vi "Workspace.Initialize.vi"(11 "State":T1) -> (0 "error out":errorcluster, 3 "State":T1)   [LabVIEW 2023, in "J1939 Workspace Shared.lvlib"]
uses:
  J1939 Workspace Shared.lvlib
  Types/UI.StateVariables.ctl
  <vilib>/NI VeriStand/Display Template Support/DisplayTemplateSupport.llb/enum_Display Template Handler Minimal To Widget Msg.ctl
  <vilib>/NI VeriStand/Execution/Workspace/SystemStateRegEventRef.ctl
  <vilib>/NI VeriStand/Execution/Workspace/Target State Info.ctl
  <vilib>/NI VeriStand/Execution/Workspace/Target State.ctl
  Types/Private Data.ctl
  <vilib>/NI/STM/TCP/TCP Connection Info.ctl
  <vilib>/NI/STM/SubVIs/MetaDataElement.ctl
  Addon/Addon Shared/Types/Error Cluster.ctl
  Addon/Addon Shared/Types/Error Types.ctl
  NationalInstruments.VeriStand.SystemStorage
  <vilib>/NI VeriStand/Display Template Support/DisplayTemplateSupport.llb/enum_Display Template Handler Minimal To Workspace.ctl
  <vilib>/NI VeriStand/Execution/Workspace/WorkspaceAPI.ctl
  NationalInstruments.VeriStand.ClientAPI
  <vilib>/NI VeriStand/Execution/Workspace/SystemStateEventRef.ctl
  Types/UI.Refs.ctl
  SubModules/CAN-Streaming-Support/Source/Addon/Addon Shared/Types/Type Filter.ctl
  SubModules/CAN-Streaming-Support/Source/Addon/Addon Shared/Types/Direction Filter.ctl
  SubModules/CAN-Streaming-Support/Source/UIs/Workspace Shared/Types/Host Stream Queue Refs.ctl
  SubModules/CAN-Streaming-Support/Source/UIs/Workspace Shared/Types/Host Stream Queue Type.ctl
  SubModules/CAN-Streaming-Support/Source/UIs/Workspace Shared/Types/Host Stream Queue Command.ctl
  <vilib>/xnet/xnet.llb/XNET Frame CAN.ctl
  <vilib>/xnet/xnet.llb/XNET Frame Type CAN.ctl
  <vilib>/NI VeriStand/Execution/Workspace/NI_VS Workspace ExecutionAPI.lvlib
  Addon/Addon Shared/J1939 Addon Shared.lvlib
  SubModules/CAN-Streaming-Support/Source/UIs/Workspace Shared/CAN Stream Support Workspace Shared.lvlib
  <vilib>/NI/STM/NI STM.lvlib
  SubModules/CAN-Streaming-Support/Source/Addon/Addon Shared/CAN Stream Support Shared.lvlib
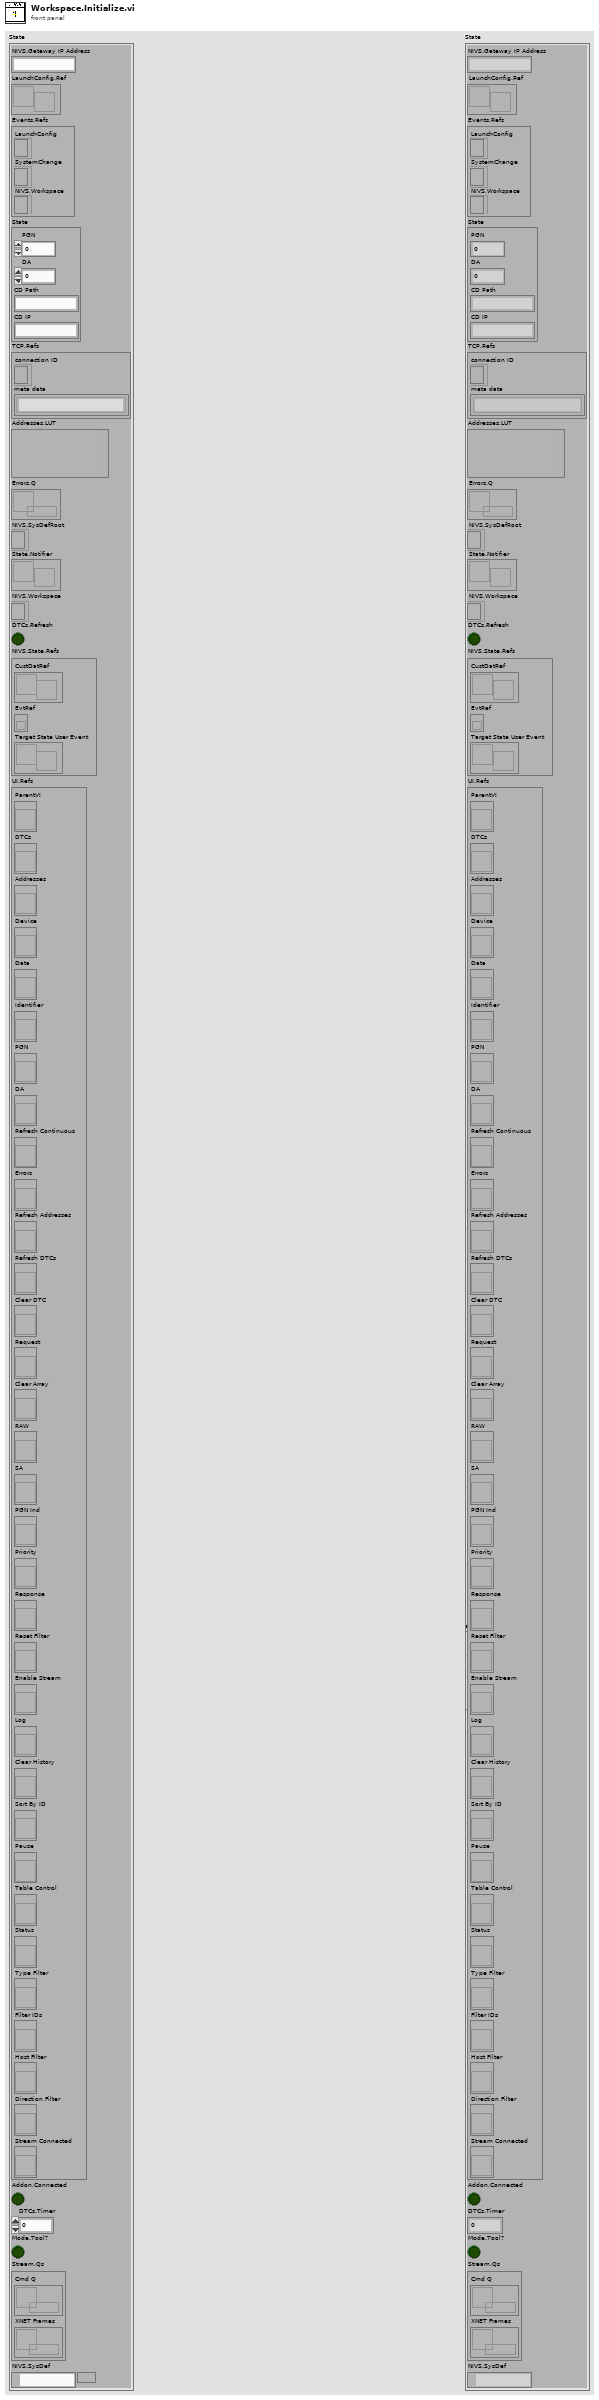
[diagram p1: front panel]
types:
  T1 = typedef "J1939 Workspace Shared.lvlib/UI.StateVariables.ctl" = cluster{"NIVS.Gateway IP Address":string, "LaunchConfig.Ref":refnum<user-event>, "Events.Refs":cluster{"LaunchConfig":refnum<event-registration>, "SystemChange":T2, "NIVS.Workspace":refnum<event-registration>}, "State":T3, "TCP.Refs":T4, "Addresses.LUT":variant, "Errors.Q":refnum<queue>, "NIVS.SysDefRoot":refnum<k24>, "State.Notifier":refnum<user-event>, "NIVS.Workspace":T6, "DTCs.Refresh":bool, "NIVS.State.Refs":T7, "UI.Refs":T8, "Addon.Connected":bool, "DTCs.Timer":u32, "Mode.Tool?":bool, "Stream.Qs":T9, "NIVS.SysDef":path}
  T2 = typedef "NI_VS Workspace ExecutionAPI.lvlib/SystemStateRegEventRef.ctl" = refnum<event-registration>
  T3 = typedef "J1939 Workspace Shared.lvlib/Private Data.ctl" = cluster{"PGN":u32, "DA":u8, "CD Path":string, "CD IP":string}
  T4 = typedef "NI STM.lvlib/TCP Connection Info.ctl" = cluster{"connection ID":refnum<k5>, "meta data":T5[]}
  T5 = typedef "NI STM.lvlib/MetaDataElement.ctl" = string
  T6 = typedef "NI_VS Workspace ExecutionAPI.lvlib/WorkspaceAPI.ctl" = refnum<k24>
  T7 = typedef "NI_VS Workspace ExecutionAPI.lvlib/SystemStateEventRef.ctl" = cluster{"CustDatRef":refnum<user-event>, "EvtRef":refnum<k27>, "Target State User Event":refnum<user-event>}
  T8 = typedef "J1939 Workspace Shared.lvlib/UI.Refs.ctl" = cluster{"ParentVI":refnum<vi>, "DTCs":refnum<vi>, "Addresses":refnum<vi>, "Device":refnum<vi>, "Data":refnum<vi>, "Identifier":refnum<vi>, "PGN":refnum<vi>, "DA":refnum<vi>, "Refresh Continuous":refnum<vi>, "Errors":refnum<vi>, "Refresh Addresses":refnum<vi>, "Refresh DTCs":refnum<vi>, "Clear DTC":refnum<vi>, "Request":refnum<vi>, "Clear Array":refnum<vi>, "RAW":refnum<vi>, "SA":refnum<vi>, "PGN Ind":refnum<vi>, "Priority":refnum<vi>, "Response":refnum<vi>, "Reset Filter":refnum<vi>, "Enable Stream":refnum<vi>, "Log":refnum<vi>, "Clear History":refnum<vi>, "Sort By ID":refnum<vi>, "Pause":refnum<vi>, "Table Control":refnum<vi>, "Status":refnum<vi>, "Type Filter":refnum<vi>, "Filter IDs":refnum<vi>, "Host Filter":refnum<vi>, "Direction Filter":refnum<vi>, "Stream Connected":refnum<vi>}
  T9 = typedef "CAN Stream Support Workspace Shared.lvlib/Host Stream Queue Refs.ctl" = cluster{"Cmd Q":refnum<queue>, "XNET Frames":refnum<queue>}
  T10 = typedef "J1939 Addon Shared.lvlib/Error Cluster.ctl" = cluster{"error out":errorcluster, "Enum":T11, "Address":u8, "Timestamp":timestamp}
  T11 = typedef "J1939 Addon Shared.lvlib/Error Types.ctl" = enum16{"Request", "RAW Generation", "Clear Active DTCs", "Clear Previous DTCs", "Addresses", "TLAs", "Get Active DTCs", "Get Previous DTCs", "TCP Connection"}
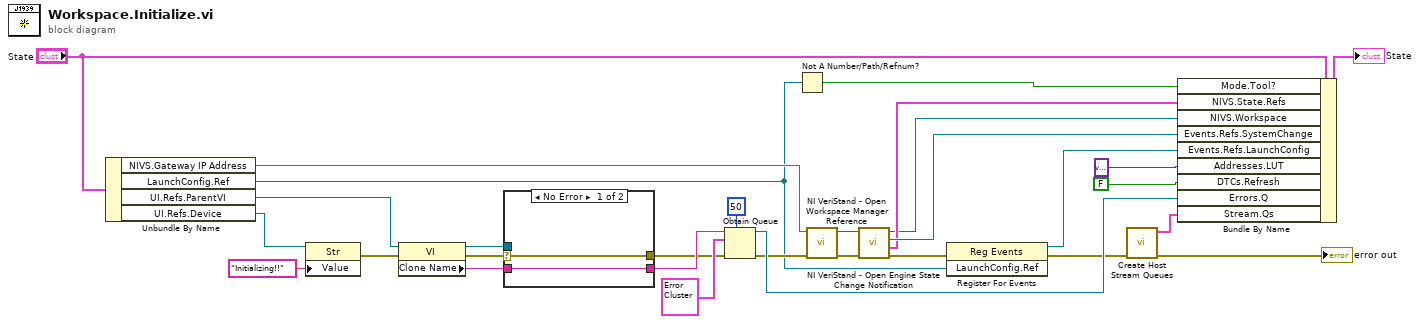
[diagram p0: block diagram]
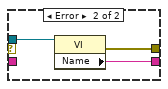
[diagram p2: hidden frame]
diagram:
  n1 = Unbundle By Name("State") -> ("NIVS.Gateway IP Address"=w19:string, "LaunchConfig.Ref"=w5:refnum<user-event>, "UI.Refs.ParentVI"=w15:refnum<vi>, "UI.Refs.Device"=w7:refnum<vi>)
  n2 = property class="Str"(reference=w7, "Value"="Initializing!!") -> (error out=w8:errorcluster)  [unwired: 1 in, 1 out]
  n3 = property class="VI"(reference=w15, error in=w8) -> (reference out=w12:refnum<vi>, error out=w13:errorcluster, "Clone Name"=w9:string)
  n4 = case shown="No Error" w13 {
    selector: w13 -> [w31 _]
    tunnel: w12 -> [_ w35]
    tunnel: [w32 w34] -> w11
    tunnel: [w31 w33] -> w10
    tunnel: w9 -> [w32 _]
    frame No Error {
    }
    frame Error {
      n5 = property class="VI"(reference=w35) -> (error out=w33:errorcluster, "Name"=w34:string)  [unwired: 1 in, 1 out]
    }
  }
  n6 = Obtain Queue(max queue size (-1, unlimited)=50, name (unnamed)=w11, element data type=T10 {"error out"={"status"=FALSE, "code"=0, "source"=""}, "Enum"=enum."Request", "Address"=0, "Timestamp"=timestamp(0 s since 1904-01-01)} ("Error Cluster"), error in (no error)=w10) -> (queue out=w30:refnum<queue>, error out=w14:errorcluster)  [unwired: 1 in, 1 out]
  n7 = Not A Number/Path/Refnum?(number/path/refnum=w5) -> (NaN/Path/Refnum?=w4:bool)
  n8 = call <vilib>:"NI VeriStand - Open Workspace Manager Reference.vi"("error in (no error)"=w14, "Gateway IP Address (\"\": localhost)"=w19) -> ("error out"=w17:errorcluster, "WorkspaceManager"=w16:T6)  [unwired: 8 in]
  n9 = call <vilib>:"NI VeriStand - Open Engine State Change Notification.vi"("error in (no error)"=w17, "WorkspaceManager in"=w16) -> ("error out"=w18:errorcluster, "SystemStateRefs"=w27:T7, "SystemChangeEventRef"=w29:T2, "WorkspaceManager out"=w21:T6)  [unwired: 6 in]
  n10 = register-events(error in=w18, w5) -> (reference out=w28:refnum<event-registration>, error out=w3:errorcluster)  [unwired: 1 in]
  n11 = call "Create Host Stream Queues.vi"("error in (no error)"=w3) -> ("error out"=→"error out":errorcluster, "Q Refs"=w1:T9)  [unwired: 9 in]
  n12 = Bundle By Name(cluster="State", "Mode.Tool?"=w4, "NIVS.State.Refs"=w27, "NIVS.Workspace"=w21, "Events.Refs.SystemChange"=w29, "Events.Refs.LaunchConfig"=w28, "Addresses.LUT"=variant ("Addresses"), "DTCs.Refresh"=FALSE, "Errors.Q"=w30, "Stream.Qs"=w1) -> (→"State":T1)
